vi "vipm_unInstallPackages.vi"(8 "error in (no error)":errorcluster, 11 "CommandLine":string[](array[string])) -> (0 "error out":errorcluster, 2 "test details":string, 3 "output to action":string)   [LabVIEW 2014]
uses:
  <userlib>/_OpenG.lib/array/array.llb/Index 1D Array Elements (String)__ogtk.vi
  <userlib>/_OpenG.lib/array/array.llb/Filter 1D Array (String)__ogtk.vi
  <vilib>/JKI/VIPM API/VIPM API_vipm_api.lvlib
  _lvcicd/_lvcicd_support_2014.lvlib
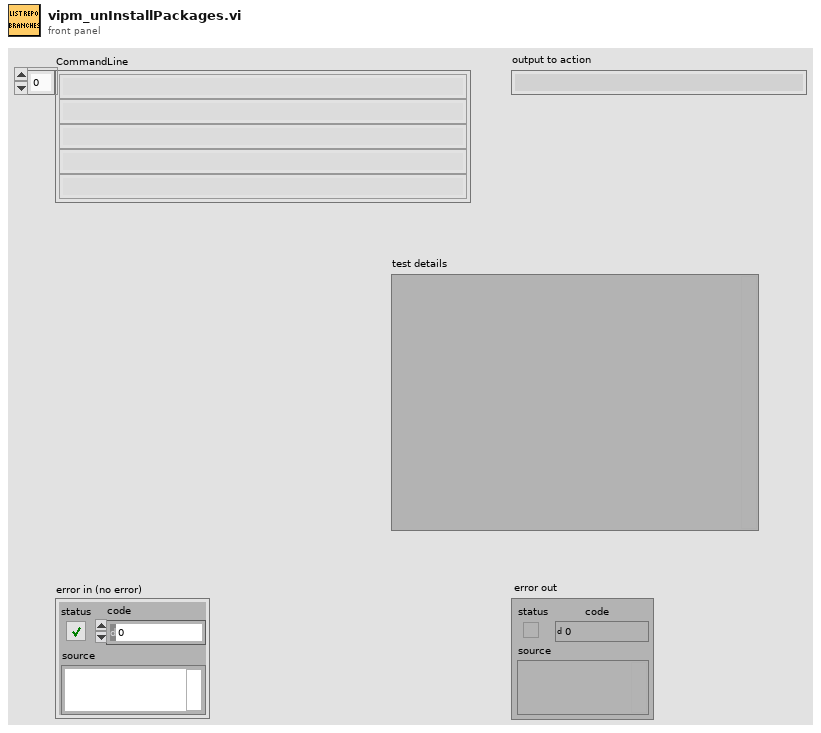
[diagram p1: front panel]
types:
  T1 = typedef "VIPM API_vipm_api.lvlib/Library Contents Cluster_vipm_api.ctl" = cluster{"Package Name":string, "Version":string, "Display Name":string, "Repository Name":string, "Company Name":string, "License Type":string, "Installed":bool, "Deprecated":bool, "Dependency or Conflict Problem":bool, "Downloaded":bool}
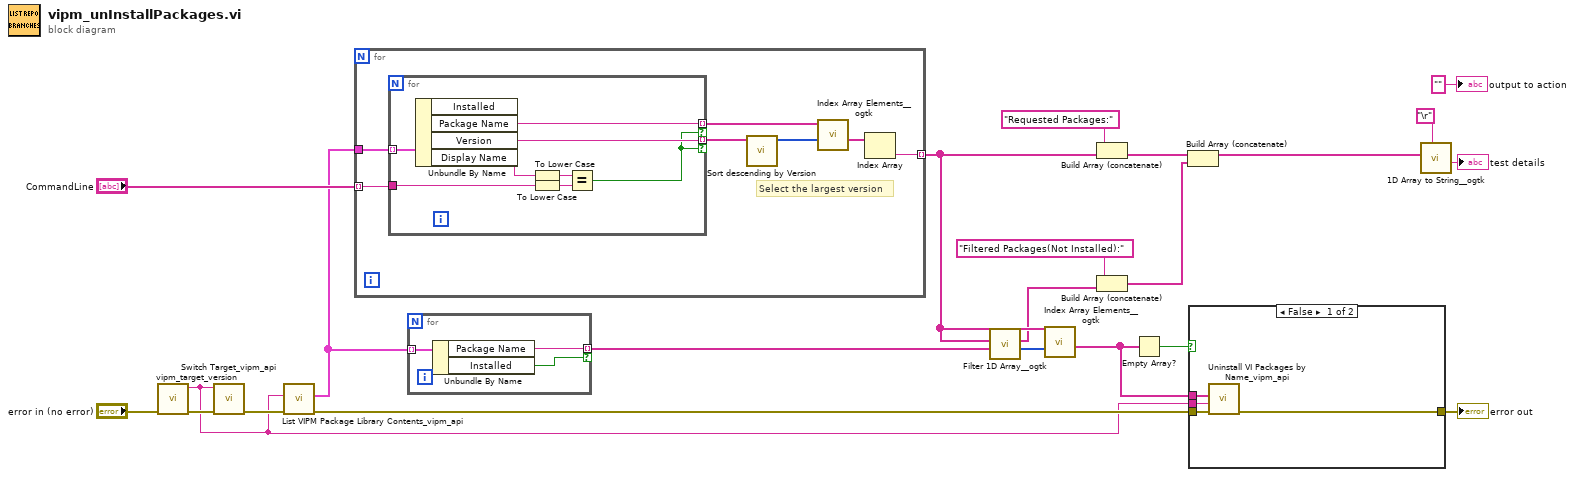
[diagram p0: block diagram]
diagram:
  n1 = call "vipm_target_version.vi"() -> ("vipm Taget version"=w14:string)  [unwired: 11 in]
  n2 = call <vilib>:"Switch Target_vipm_api.vi"("error in (no error)"="error in (no error)", "LabVIEW Version"=w14) -> ("error out"=w15:errorcluster)  [unwired: 9 in]
  n3 = call <vilib>:"List VIPM Package Library Contents_vipm_api.vi"("error in (no error)"=w15, "LabVIEW Version"=w14) -> ("error out"=w18:errorcluster, "Library Contents []"=w12:T1[])  [unwired: 7 in, 1 out]
  n4 = for {
    tunnel: w12 -> [w28]
    tunnel: "CommandLine" -> [w27] mode=indexing
    tunnel: [w22] -> w9 mode=indexing
    # "Select the largest version"
    n5 = for {
      tunnel: w28 -> [w36] mode=indexing
      tunnel: w27 -> [w34]
      tunnel: [w33] -> w26 mode=indexing if=w31
      tunnel: [w32] -> w25 mode=indexing if=w31
      n6 = Unbundle By Name(w36) -> ("Package Name"=w32:string, "Version"=w33:string, "Display Name"=w35:string)  [unwired: 1 out]
      n7 = To Lower Case(string=w35) -> (all lower case string=w30:string)
      n8 = To Lower Case(string=w34) -> (all lower case string=w29:string)
      n9 = Equal?(x=w30, y=w29) -> (x = y?=w31:bool)
    }
    n10 = call "Sort descending by Version.vi"("Array"=w26) -> ("Sorted Pointers"=w24:i32[])  [unwired: 10 in]
    n11 = call-poly <userlib>:"Index Array Elements__ogtk.vi"("indices"=w24, "array"=w25) -> ("elements"=w23:string[])  [unwired: 9 in]
    n12 = Index Array(array=w23) -> (element=w22:string)  [unwired: 1 in]
  }
  n13 = for {
    tunnel: w12 -> [w39] mode=indexing
    tunnel: [w38] -> w11 mode=indexing if=w37
    n14 = Unbundle By Name(w39) -> ("Package Name"=w38:string, "Installed"=w37:bool)
  }
  n15 = call-poly <userlib>:"Filter 1D Array__ogtk.vi"("items to filter"=w11, "array"=w9) -> ("filtered item indices"=w10:i32[], "filtered array"=w5:string[])  [unwired: 4 in]
  n16 = call-poly <userlib>:"Index Array Elements__ogtk.vi"("indices"=w10, "array"=w9) -> ("elements"=w2:string[])  [unwired: 9 in]
  n17 = Build Array (concatenate)("Requested Packages:" ("output to action"), w9) -> (w8:string[])
  n18 = Build Array (concatenate)("Filtered Packages(Not Installed):" ("output to action"), w5) -> (w3:string[])
  n19 = Empty Array?(array=w2) -> (empty?=w1:bool)
  n20 = Build Array (concatenate)(w8, w3) -> (w4:string[])
  n21 = case shown="False" w1 {
    tunnel: [w43 w44] -> w21
    tunnel: w18 -> [w42 w44]
    tunnel: w14 -> [w41 _]
    tunnel: w2 -> [w40 _]
    frame False {
      n22 = call <vilib>:"Uninstall VI Packages by Name_vipm_api.vi"("error in (no error)"=w42, "LabVIEW Version"=w41, "Package Names to Uninstall []"=w40) -> ("error out"=w43:errorcluster)  [unwired: 8 in]
    }
    frame True {
    }
  }
  "error out" <- w21
  n23 = call <userlib>:"1D Array to String__ogtk.vi"("delimiter (Tab)"="\r", "Array of Strings"=w4) -> ("delimited string"=→"test details":string)  [unwired: 9 in]
  "output to action" <- "" ("output to action")
